vi "Normalize.vi"(8 "error in (no error)":errorcluster, 10 "eval":dbl, 11 "Objective in":refnum<class "Objective.lvclass">) -> (0 "error out":errorcluster, 2 "normalizedEval":dbl, 3 "Objective out":refnum<class "Objective.lvclass">)   [LabVIEW 2023, in "Objective.lvclass"]
uses:
  Objective.lvclass
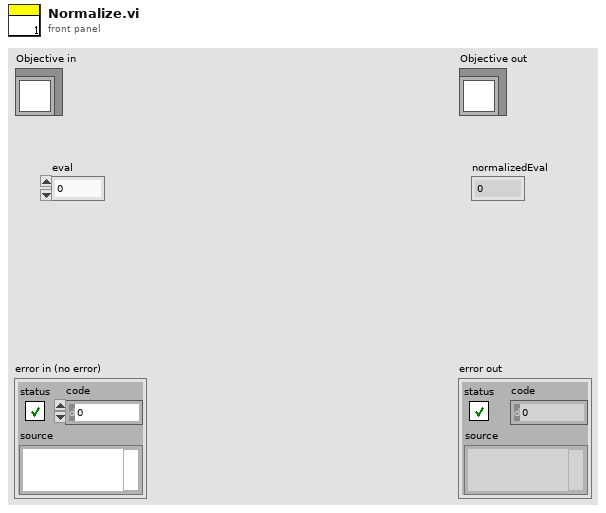
[diagram p1: front panel]
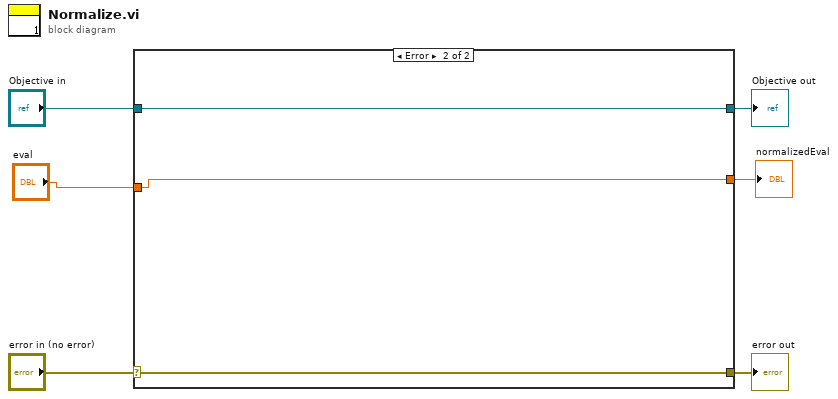
[diagram p0: block diagram]
diagram:
  n1 = case shown="Error" "error in (no error)" {
    selector: "error in (no error)" -> [w8 w12]
    tunnel: [w8 w12] -> w5
    tunnel: [w9 w11] -> w3
    tunnel: "Objective in" -> [w9 w11]
    tunnel: "eval" -> [w7 w10]
    tunnel: [w7 w10] -> w1
    frame No Error {
      # "Wire the error cluster across even in the \"No Error\"\ncase so that warnings get propagated."
    }
    frame Error {
    }
  }
  "error out" <- w5
  "Objective out" <- w3
  "normalizedEval" <- w1
